vi "Verify with Nested Scrubbers.vi"(8 "error in":errorcluster) -> (0 "error out":errorcluster)   [LabVIEW 2020, in "Scrubber.Tests.lvclass"]
uses:
  Scrubber.Tests.lvclass
  Source/Approval Tests/Options/Options.lvclass
  Source/Approval Tests/Regex Scrubber/Regex Scrubber.lvclass
  C:/Users/SAS/Desktop/ApprovalTests.LabVIEW/Source/Approval Tests/Scrubber/Scrubber.lvclass
  Source/Approval Tests/Multi Scrubber/Multi Scrubber.lvclass
  Source/Approval Tests/Regex Scrubber/Regex Scrubber.lvclass/Regex Scrubber.ctl
  Source/Approval Tests/Multi Scrubber/Multi Scrubber.lvclass/Multi Scrubber.ctl
  Source/Approval Tests/Options/Options.lvclass/Options.ctl
  Source/Approval Tests/Naming Data/Naming Data.lvclass/Naming Data.ctl
  4b862e9e-fcb2-487f-ab73-d9f83fbf4d2c.vi
  Source/Approval Tests/Regex Scrubber/Write Regex.vi
  Source/Approval Tests/Regex Scrubber/Write Replacement.vi
  Source/Approval Tests/Multi Scrubber/Write Scrubbers.vi
  Source/Approval Tests/Options/Write Set Scrubber.vi
  4b862e9e-fcb2-487f-ab73-d9f83fbf4d2c.vi/500b534b-d6f0-4fa5-90b2-c40158375321.vi
  Source/Approval Tests/Update Test Name if Not Defined.vi
  4b862e9e-fcb2-487f-ab73-d9f83fbf4d2c.vi/500b534b-d6f0-4fa5-90b2-c40158375321.vi/93c5622b-9fb7-41e0-8c76-3fde37e94e34.vi
  Source/Approval Tests/Verify Core.vi
  Source/Approval Tests/Options/Read Scrubber.vi
  Source/Approval Tests/Naming Data/Read Test VI Name.vi
  Source/Approval Tests/Naming Data/Write Test VI Name.vi
  4b862e9e-fcb2-487f-ab73-d9f83fbf4d2c.vi/500b534b-d6f0-4fa5-90b2-c40158375321.vi/93c5622b-9fb7-41e0-8c76-3fde37e94e34.vi/04cb982b-2eda-40d0-8d7e-90f8e0b569b2.vi
  Source/Approval Tests/Options/Read Namer.vi
  Source/Approval Tests/Options/Read Naming Data.vi
  Source/Approval Tests/Options/Read Reporter.vi
  Source/Approval Tests/conv EOL.vi
  <vilib>/Utility/libraryn.llb/Check if File or Folder Exists.vi
  Source/Approval Tests/Reporter/Report.vi
  <vilib>/addons/_JKI Toolkits/Caraya/classes/Assert/Assert.vi
  <vilib>/addons/_JKI Toolkits/Caraya/classes/Assert/Assert True.vi
  Source/Approval Tests/Scrubber/Scrubber.lvclass
  Source/Approval Tests/Namer/Namer.lvclass
  Source/Approval Tests/Naming Data/Naming Data.lvclass
  Source/Approval Tests/Reporter/Reporter.lvclass
  Scrubber.Tests.lvclass/Scrubber.Tests.ctl
  <vilib>/addons/_JKI Toolkits/Caraya/classes/Test/Test.lvclass
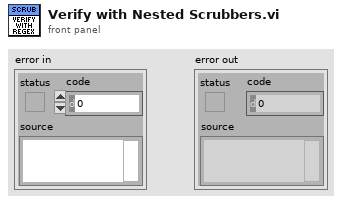
[diagram p1: front panel]
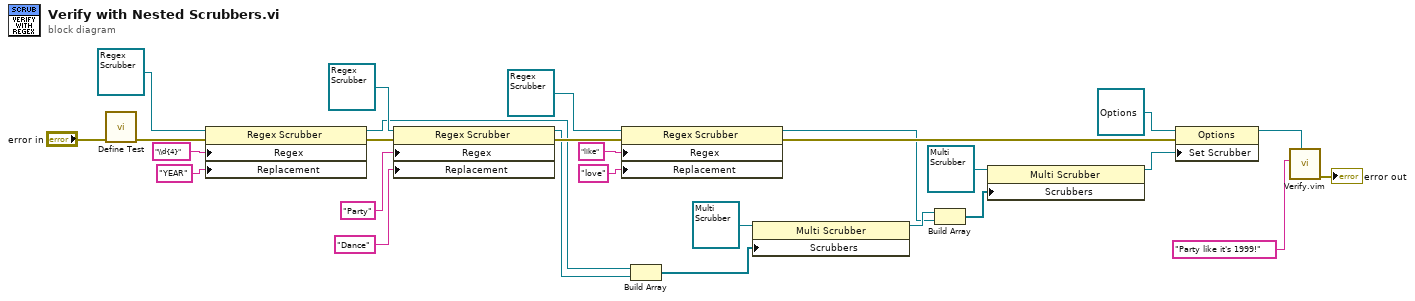
[diagram p0: block diagram]
diagram:
  n1 = call <vilib>:"Define Test.vi"("error in (no error)"="error in") -> ("error out"=w27:errorcluster)  [unwired: 9 in, 1 out]
  n2 = property class="Regex Scrubber"(reference=refnum<class "Regex Scrubber.lvclass"> refnum ("Approval Tests.lvlib:Regex Scrubber.lvclass"), error in=w27, "Regex"="\\d{4}", "Replacement"="YEAR") -> (reference out=w7:refnum<class "Regex Scrubber.lvclass">, error out=w24:errorcluster)
  n3 = property class="Regex Scrubber"(reference=refnum<class "Regex Scrubber.lvclass"> refnum ("Approval Tests.lvlib:Regex Scrubber.lvclass"), error in=w24, "Regex"="Party", "Replacement"="Dance") -> (reference out=w6:refnum<class "Regex Scrubber.lvclass">, error out=w23:errorcluster)
  n4 = property class="Regex Scrubber"(reference=refnum<class "Regex Scrubber.lvclass"> refnum ("Approval Tests.lvlib:Regex Scrubber.lvclass"), error in=w23, "Regex"="like", "Replacement"="love") -> (reference out=w3:refnum<class "Regex Scrubber.lvclass">, error out=w22:errorcluster)
  n5 = Build Array(w7, w6) -> (w5:refnum<class "Regex Scrubber.lvclass">[])
  n6 = property class="Multi Scrubber"(reference=refnum<class "Multi Scrubber.lvclass"> refnum ("Approval Tests.lvlib:Multi Scrubber.lvclass"), "Scrubbers"=w5) -> (reference out=w4:refnum<class "Multi Scrubber.lvclass">)  [unwired: 1 in, 1 out]
  n7 = Build Array(w4, w3) -> (w2:refnum<class "Scrubber.lvclass">[])
  n8 = property class="Multi Scrubber"(reference=refnum<class "Multi Scrubber.lvclass"> refnum ("Approval Tests.lvlib:Multi Scrubber.lvclass"), "Scrubbers"=w2) -> (reference out=w1:refnum<class "Multi Scrubber.lvclass">)  [unwired: 1 in, 1 out]
  n9 = property class="Options"(reference=refnum<class "Options.lvclass"> refnum ("Approval Tests.lvlib:Options.lvclass"), error in=w22, "Set Scrubber"=w1) -> (reference out=w8:refnum<class "Options.lvclass">)  [unwired: 1 out]
  n10 = call "Verify.vim"("Options"=w8, "Test Data"="Party like it's 1999!") -> ("error out"=→"error out":errorcluster)  [unwired: 8 in, 1 out]
